vi "Transpose 2D Array.vi"() -> ()   [LabVIEW 2019]
panel:
  in  "InnerLoop Output  2":dbl[][](array[numeric])
  out "output array":dbl[](array[numeric])
  out "InnerLoop Output":dbl[][](array[numeric])
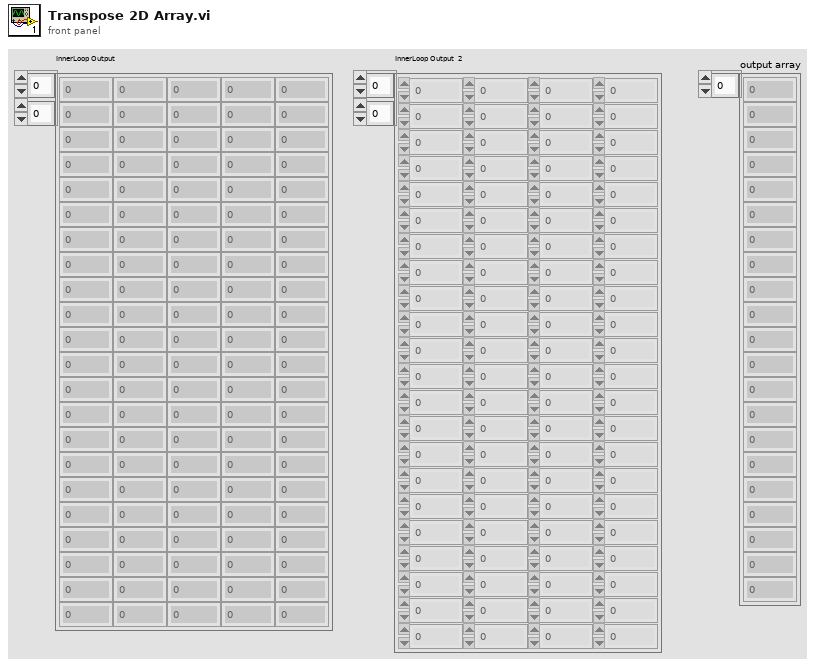
[diagram p1: front panel]
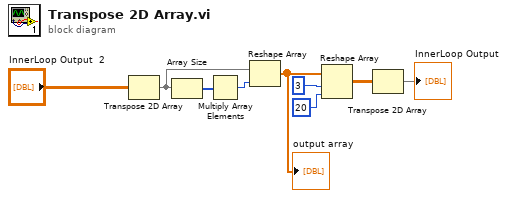
[diagram p0: block diagram]
diagram:
  n1 = Transpose 2D Array(2D array="InnerLoop Output  2") -> (transposed array=w2:dbl[][])
  n2 = Array Size(array=w2) -> (size(s)=w6:i32[])
  n3 = Multiply Array Elements(1:w6) -> (0:w5:i32)
  n4 = Reshape Array(w2, w5) -> (w1:dbl[])
  "output array" <- w1
  n5 = Reshape Array(w1, 3 ("dimension size"), 20 ("dimension size")) -> (w7:dbl[][])
  n6 = Transpose 2D Array(2D array=w7) -> (transposed array=→"InnerLoop Output":dbl[][])
